vi "SLSC Get Default-Reset Value.vi"(8 "error in (no error)":errorcluster, 11 "Section Ref in":T1 format="%.0x") -> (0 "error out":errorcluster, 1 "Apply Reset":bool, 2 "Apply Default":bool, 3 "Item Ref out":T1 format="%.0x")   [LabVIEW 2015, in "SLSC EDS System Explorer.lvlib"]
uses:
  System Explorer/SLSC EDS System Explorer.lvlib
  <vilib>/NI Veristand/Custom Device API/Custom Device Item Ref.ctl
  Shared/Constants.vi
  <vilib>/NI Veristand/Custom Device API/Get Item Property (Boolean).vi
  Shared/SLSC EDS Shared.lvlib
  <vilib>/NI VeriStand/Custom Device API/Custom Device API.lvlib
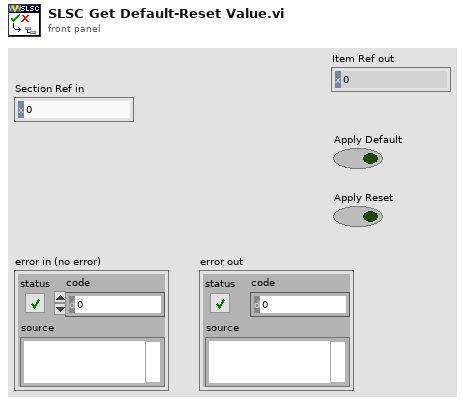
[diagram p1: front panel]
types:
  T1 = typedef "Custom Device API.lvlib/Custom Device Item Ref.ctl" = u64
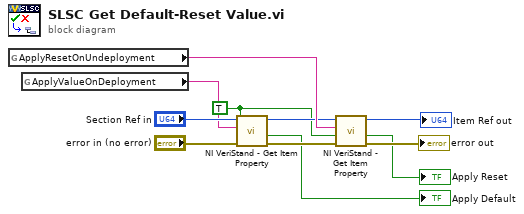
[diagram p0: block diagram]
diagram:
  w1 = TRUE ("Default Value")
  n1 = global read "Constants.vi" "ApplyResetOnUndeployment"() -> (w7:string)
  n2 = global read "Constants.vi" "ApplyValueOnDeployment"() -> (w5:string)
  n3 = call-poly <vilib>:"NI VeriStand - Get Item Property.vi"("error in (no error)"="error in (no error)", "Default Value"=w1, "Property Name"=w5, "Item Ref in"="Section Ref in") -> ("error out"=w10:errorcluster, "Value"=→"Apply Default":bool, "Item Ref out"=w6:T1)  [unwired: 4 in, 1 out]
  n4 = call-poly <vilib>:"NI VeriStand - Get Item Property.vi"("error in (no error)"=w10, "Default Value"=w1, "Property Name"=w7, "Item Ref in"=w6) -> ("error out"=→"error out":errorcluster, "Value"=→"Apply Reset":bool, "Item Ref out"=→"Item Ref out":T1)  [unwired: 4 in, 1 out]
